vi "ma_sml_Peak Rough Search Indices (advanced).vi"(0 "spectrum":T2={"f0"=1.0, "df"=1.0, "spectrum"=[]} {"spectrum" format="%.2f"; "df" format="%.2f"; "f0" format="%.2f"}, 1 "peak search mode":u16(ring) items=["Threshold", "Highest N Peaks", "Peaks Near Frequencies"], 2 "threshold":dbl format="%.2f", 3 "highest n peaks":i32=1, 4 "peaks near frequencies":T1={"frequencies"=[], "tolerance (Hz)"=100.0} {"tolerance (Hz)" format="%_4p"; "frequencies" format="%_4p"}) -> (5 "peak indices":i32[](array[numeric]))   [LabVIEW 2020, in "NI_MAPro.lvlib"]
uses:
  NI_MAPro.lvlib
  ma_sml_Spectrum Cluster (real).ctl
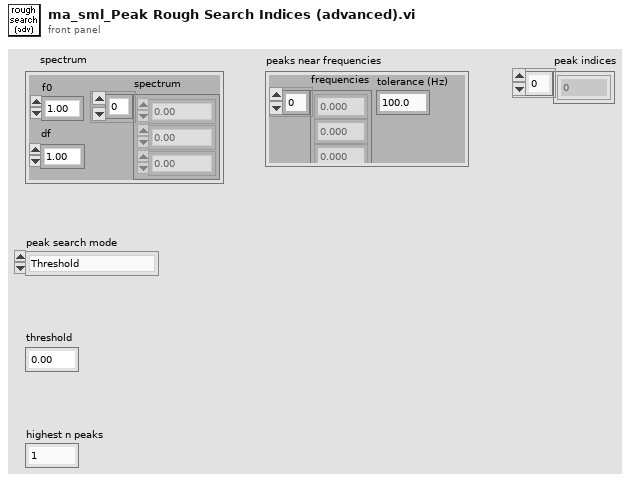
[diagram p1: front panel]
types:
  T1 = cluster{"frequencies":dbl[], "tolerance (Hz)":dbl}
  T2 = typedef "NI_MAPro.lvlib/ma_sml_Spectrum Cluster (real).ctl" = cluster{"f0":dbl, "df":dbl, "spectrum":dbl[]}
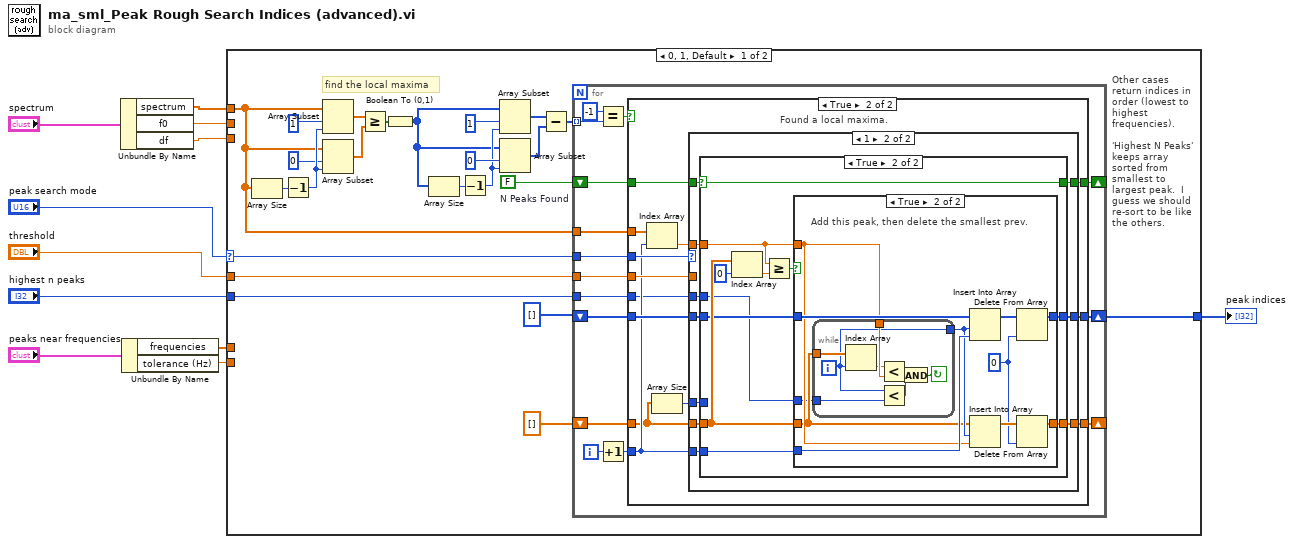
[diagram p0: block diagram]
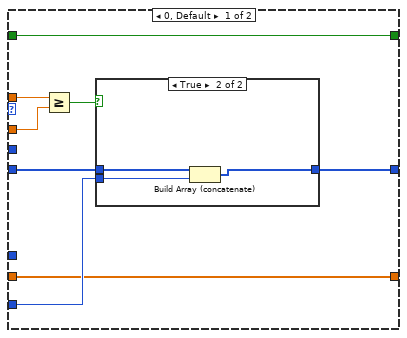
[diagram p3: hidden frame]
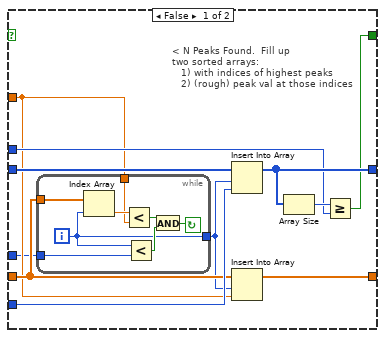
[diagram p5: hidden frame]
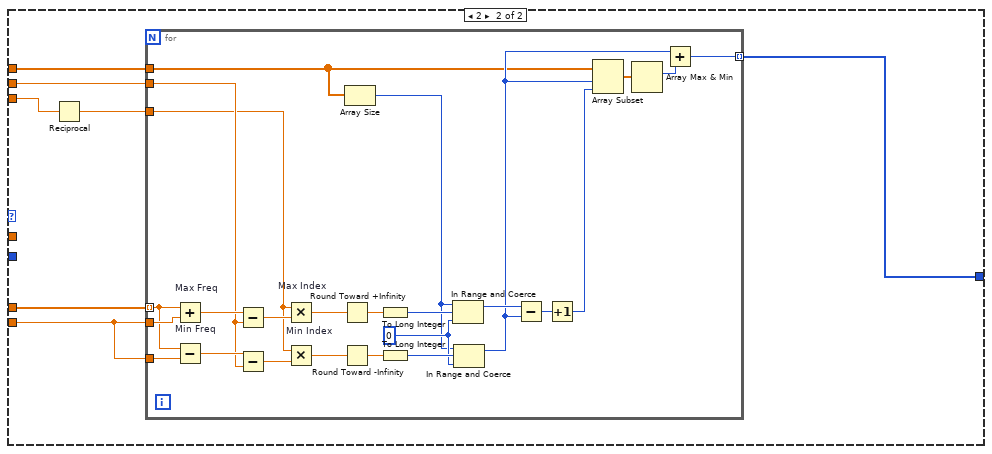
[diagram p7: hidden frame]
diagram:
  n1 = Unbundle By Name("spectrum") -> ("spectrum"=w2:dbl[], "f0"=w4:dbl, "df"=w3:dbl)
  n2 = Unbundle By Name("peaks near frequencies") -> ("frequencies"=w11:dbl[], "tolerance (Hz)"=w10:dbl)
  n3 = case shown="0, 1, Default" "peak search mode" {
    selector: "peak search mode" -> [w30 _]
    tunnel: [w13 w139] -> w1
    tunnel: w2 -> [w12 w141]
    tunnel: "threshold" -> [w34 _]
    tunnel: w11 -> [_ w145]
    tunnel: w10 -> [_ w140]
    tunnel: w3 -> [_ w143]
    tunnel: w4 -> [_ w144]
    tunnel: "highest n peaks" -> [w29 _]
    frame 0, 1, Default {
      w31 = FALSE  # N Peaks Found
      # "find the local maxima"
      # "Other cases return indices in order (lowest to highest frequencies).  \n\n'Highest N Peaks' keeps array sorted from smallest to largest peak.  I guess we should re-sort to be like the others."
      n4 = Array Size(array=w12) -> (size(s)=w27:i32)
      n5 = Decrement(x=w27) -> (x-1=w26:i32)
      n6 = Array Subset(array=w12, index=1, length=w26) -> (w23:dbl[])
      n7 = Array Subset(array=w12, index=0, length=w26) -> (w22:dbl[])
      n8 = Greater Or Equal?(x=w23, y=w22) -> (x >= y?=w21:bool[])
      n9 = Boolean To (0,1)(Boolean=w21) -> (0, 1=w16:i16[])
      n10 = Array Size(array=w16) -> (size(s)=w17:i32)
      n11 = Decrement(x=w17) -> (x-1=w18:i32)
      n12 = Array Subset(array=w16, index=1, length=w18) -> (w15:i16[])
      n13 = Array Subset(array=w16, index=0, length=w18) -> (w14:i16[])
      n14 = Subtract(x=w15, y=w14) -> (x-y=w28:i16[])
      n15 = for {
        shift-right: [w46] -> w13
        shift-left: i32[] [] -> [w47]
        tunnel: w28 -> [w36] mode=indexing
        tunnel: w12 -> [w49]
        tunnel: w34 -> [w48]
        tunnel: w30 -> [w43]
        shift-right: [w40] -> _
        shift-left: dbl[] [] -> [w42]
        shift-right: [w39] -> _
        shift-left: w31 -> [w41]
        tunnel: w29 -> [w38]
        i -> [w45]
        n16 = Equal?(x=i16 -1, y=w36) -> (x = y?=w35:bool)
        n17 = Increment(x=w45) -> (x+1=w44:i32)
        n18 = case shown="True" w35 {
          tunnel: w49 -> [_ w59]
          tunnel: w48 -> [_ w65]
          tunnel: w47 -> [w52 w64]
          tunnel: [w52 w63] -> w46
          tunnel: w44 -> [_ w58]
          tunnel: w43 -> [_ w62]
          tunnel: w42 -> [w51 w54]
          tunnel: w41 -> [w50 w61]
          tunnel: [w51 w60] -> w40
          tunnel: [w50 w56] -> w39
          tunnel: w38 -> [_ w55]
          frame False {
          }
          frame True {
            # "Found a local maxima."
            n19 = Index Array(array=w59, index=w58) -> (element=w57:dbl)
            n20 = Array Size(array=w54) -> (size(s)=w53:i32)
            n21 = case shown="1" w62 {
              tunnel: w65 -> [w73 _]
              tunnel: w64 -> [w72 w84]
              tunnel: [w71 w82] -> w63
              tunnel: w58 -> [w70 w87]
              tunnel: w54 -> [w67 w85]
              tunnel: w61 -> [w66 w86]
              tunnel: [w67 w83] -> w60
              tunnel: w57 -> [w68 w81]
              tunnel: [w66 w80] -> w56
              tunnel: w55 -> [_ w79]
              tunnel: w53 -> [_ w78]
              frame 0, Default {
                n22 = Greater Or Equal?(x=w68, y=w73) -> (x >= y?=w69:bool)
                n23 = case shown="True" w69 {
                  tunnel: w70 -> [_ w77]
                  tunnel: w72 -> [w74 w76]
                  tunnel: [w74 w75] -> w71
                  frame False {
                  }
                  frame True {
                    n24 = Build Array (concatenate)(w76, w77) -> (w75:i32[])
                  }
                }
              }
              frame 1 {
                n25 = case shown="True" w86 {
                  selector: w86 -> [_ w110]
                  tunnel: w87 -> [w93 w109]
                  tunnel: w85 -> [w91 w115]
                  tunnel: w84 -> [w98 w114]
                  tunnel: [w97 w113] -> w83
                  tunnel: [w96 w112] -> w82
                  tunnel: w81 -> [w90 w111]
                  tunnel: [w94 w110] -> w80
                  tunnel: w79 -> [w92 w107]
                  tunnel: w78 -> [w88 _]
                  frame False {
                    # "< N Peaks Found.  Fill up\ntwo sorted arrays:\n   1) with indices of highest peaks\n   2) (rough) peak val at those indices"
                    n26 = while {
                      tunnel: w91 -> [w104]
                      tunnel: w90 -> [w105]
                      tunnel: [w100] -> w89
                      tunnel: w88 -> [w99]
                      i -> [w100]
                      stop <- w102 continue-if-true
                      n27 = Index Array(array=w104, index=w100) -> (element=w106:dbl)
                      n28 = Less?(x=w106, y=w105) -> (x < y?=w101:bool)
                      n29 = Less?(x=w100, y=w99) -> (x < y?=w103:bool)
                      n30 = And(x=w101, y=w103) -> (x .and. y?=w102:bool)
                    }
                    n31 = Insert Into Array(array=w98, index=w89, new element=w93) -> (w96:i32[])
                    n32 = Insert Into Array(array=w91, index=w89, new element=w90) -> (w97:dbl[])
                    n33 = Array Size(array=w96) -> (size(s)=w95:i32)
                    n34 = Greater Or Equal?(x=w95, y=w92) -> (x >= y?=w94:bool)
                  }
                  frame True {
                    n35 = Index Array(array=w115, index=0) -> (element=w117:dbl)
                    n36 = Greater Or Equal?(x=w111, y=w117) -> (x >= y?=w116:bool)
                    n37 = case shown="True" w116 {
                      tunnel: w115 -> [w118 w121]
                      tunnel: w111 -> [_ w123]
                      tunnel: w114 -> [w119 w130]
                      tunnel: [w118 w127] -> w113
                      tunnel: [w119 w126] -> w112
                      tunnel: w109 -> [_ w125]
                      tunnel: w107 -> [_ w120]
                      frame False {
                        # "No need to add this peak.  It is smaller than the 'N' we already have."
                      }
                      frame True {
                        w124 = 0 ("index")
                        # "Add this peak, then delete the smallest prev."
                        n38 = while {
                          tunnel: w121 -> [w138]
                          tunnel: w123 -> [w137]
                          tunnel: [w135] -> w122
                          tunnel: w120 -> [w134]
                          i -> [w135]
                          stop <- w131 continue-if-true
                          n39 = Index Array(array=w138, index=w135) -> (element=w136:dbl)
                          n40 = Less?(x=w136, y=w137) -> (x < y?=w133:bool)
                          n41 = Less?(x=w135, y=w134) -> (x < y?=w132:bool)
                          n42 = And(x=w133, y=w132) -> (x .and. y?=w131:bool)
                        }
                        n43 = Insert Into Array(array=w130, index=w122, new element=w125) -> (w129:i32[])
                        n44 = Insert Into Array(array=w121, index=w122, new element=w123) -> (w128:dbl[])
                        n45 = Delete From Array(array=w129, index=w124) -> (array with subset deleted=w126:i32[])  [unwired: 1 in, 1 out]
                        n46 = Delete From Array(array=w128, index=w124) -> (array with subset deleted=w127:dbl[])  [unwired: 1 in, 1 out]
                      }
                    }
                  }
                }
              }
            }
          }
        }
      }
    }
    frame 2 {
      n47 = Reciprocal(x=w143) -> (1/x=w142:dbl)
      n48 = for {
        tunnel: w140 -> [w170]
        tunnel: w140 -> [w168]
        tunnel: w145 -> [w169] mode=indexing
        tunnel: w144 -> [w165]
        tunnel: w142 -> [w162]
        tunnel: w141 -> [w147]
        tunnel: [w153] -> w139 mode=indexing
        w148 = 0 ("lower limit")
        n49 = Add "Max Freq"(x=w169, y=w170) -> (x+y=w167:dbl)
        n50 = Subtract "Min Freq"(x=w169, y=w168) -> (x-y=w166:dbl)
        n51 = Subtract(x=w167, y=w165) -> (x-y=w164:dbl)
        n52 = Subtract(x=w166, y=w165) -> (x-y=w163:dbl)
        n53 = Multiply "Max Index"(x=w162, y=w164) -> (x*y=w157:dbl)
        n54 = Multiply "Min Index"(x=w162, y=w163) -> (x*y=w159:dbl)
        n55 = Round Toward +Infinity(x=w157) -> (ceil(x): smallest int >= x=w156:dbl)
        n56 = Round Toward -Infinity(1:w159) -> (0:w158:dbl)
        n57 = Array Size(array=w147) -> (size(s)=w146:i32)
        n58 = To Long Integer(number=w156) -> (32bit integer=w152:i32)
        n59 = To Long Integer(number=w158) -> (32bit integer=w150:i32)
        n60 = In Range and Coerce(upper limit=w146, x=w152, lower limit=w148) -> (coerced(x)=w151:i32)  [unwired: 1 out]
        n61 = In Range and Coerce(upper limit=w146, x=w150, lower limit=w148) -> (coerced(x)=w149:i32)  [unwired: 1 out]
        n62 = Subtract(x=w151, y=w149) -> (x-y=w160:i32)
        n63 = Increment(x=w160) -> (x+1=w155:i32)
        n64 = Array Subset(array=w147, index=w149, length=w155) -> (w161:dbl[])
        n65 = Array Max & Min(array=w161) -> (max index (indices)=w154:i32)  [unwired: 3 out]
        n66 = Add(x=w149, y=w154) -> (x+y=w153:i32)
      }
    }
  }
  "peak indices" <- w1
